vi "Scratch.vi"() -> ()   [LabVIEW 2015]
panel:
  in  "Cluster":T1
  out "JSON string":string
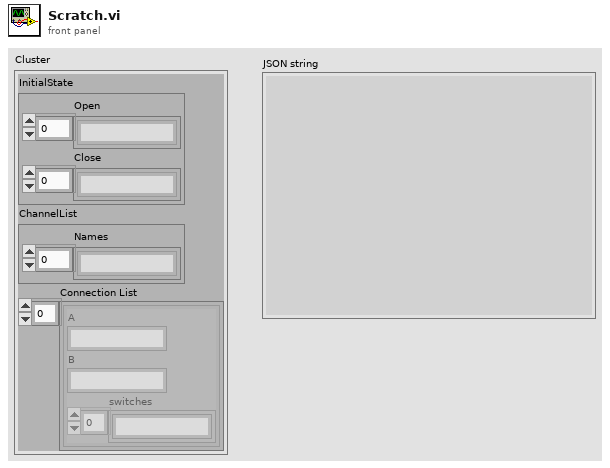
[diagram p1: front panel]
types:
  T1 = cluster{"InitialState":cluster{"Open":string[], "Close":string[]}, "ChannelList":cluster{"Names":string[]}, "Connection List":cluster{"A":string, "B":string, "switches":string[]}[]}
  T2 = cluster{"A":string, "B":string, "switches":string[]}
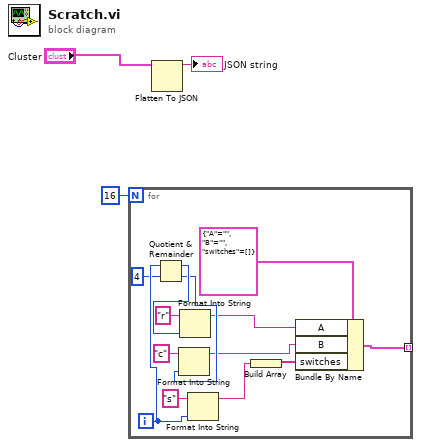
[diagram p0: block diagram]
diagram:
  n1 = for {
    N: 16 -> [_]
    tunnel: [w4] -> _ mode=indexing
    i -> [w10]
    n2 = Quotient & Remainder(x=w10, y=4) -> (x-y*floor(x/y)=w8:i32, floor(x/y)=w7:i32)
    n3 = Format Into String(initial string="c", w7) -> (resulting string=w5:string)  [unwired: 2 in, 1 out]
    n4 = Format Into String(initial string="r", w8) -> (resulting string=w6:string)  [unwired: 2 in, 1 out]
    n5 = Format Into String(initial string="s", w10) -> (resulting string=w15:string)  [unwired: 2 in, 1 out]
    n6 = Build Array(w15) -> (w14:string[])
    n7 = Bundle By Name(cluster=T2 {"A"="", "B"="", "switches"=[]} ("Cluster 2"), "A"=w6, "B"=w5, "switches"=w14) -> (w4:T2)
  }
  n8 = Flatten To JSON(anything="Cluster") -> (JSON string=→"JSON string":string)  [unwired: 2 in, 1 out]
